vi "GetVIRef.vi"(10 "CallMode":T1, 11 "CommandVI":string) -> (0 "ErrorOut":errorcluster, 3 "VIOut":refnum<vi>)   [LabVIEW 2021, in "YActor.lvclass"]
uses:
  YActor.lvclass
  CallMode.ctl
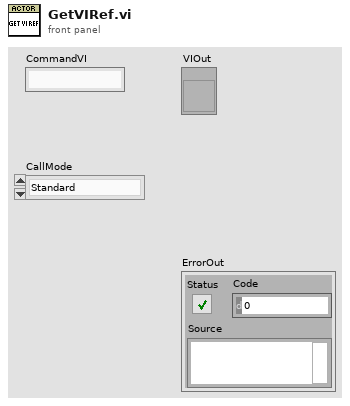
[diagram p1: front panel]
types:
  T1 = typedef "YActor.lvclass/CallMode.ctl" = enum16{"Standard", "Call&Collect"}
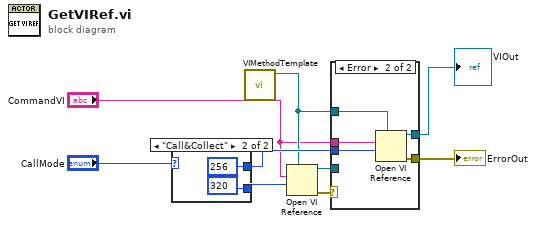
[diagram p0: block diagram]
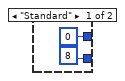
[diagram p2: hidden frame]
diagram:
  n1 = case shown="\"Call&Collect\"" "CallMode" {
    tunnel: [8 ("options") 320 ("options")] -> w6
    tunnel: [0 ("options") 256 ("options")] -> w7
    frame "Standard" {
    }
    frame "Call&Collect" {
    }
  }
  n2 = call "VIMethodTemplate.vi"() -> ("VIOut"=w2:refnum<vi>)  [unwired: 11 in]
  n3 = Open VI Reference(type specifier VI Refnum (for type only)=w2, vi path="CommandVI", options=w6) -> (vi reference=w4:refnum<vi>, error out=w8:errorcluster)  [unwired: 3 in]
  n4 = case shown="Error" w8 {
    selector: w8 -> [w15 _]
    tunnel: "CommandVI" -> [_ w19]
    tunnel: w2 -> [_ w18]
    tunnel: [w14 w17] -> w3
    tunnel: [w15 w20] -> w9
    tunnel: w4 -> [w14 _]
    tunnel: w7 -> [_ w16]
    frame No Error {
    }
    frame Error {
      n5 = Open VI Reference(type specifier VI Refnum (for type only)=w18, vi path=w19, options=w16) -> (vi reference=w17:refnum<vi>, error out=w20:errorcluster)  [unwired: 3 in]
    }
  }
  "ErrorOut" <- w9
  "VIOut" <- w3
